vi "Process.vi"(8 "error in (no error)":errorcluster, 10 "Pound in":refnum<class "Pound.lvclass">, 11 "Qbus in":refnum<class "Qbus.lvclass">) -> (0 "error out":errorcluster)   [LabVIEW 2017, in "IrManageCameras.lvlib"]
uses:
  <vilib>/addons/InsightCM/Devices/Shared/Ir/IrManageCameras/IrManageCameras.lvlib
  <vilib>/addons/Qbus/Qbus.lvclass
  <vilib>/NI/Software Watchdog/Pound/Pound.lvclass
  <vilib>/addons/InsightCM/Devices/Shared/Ir/IrManageCameras/controls/config.ctl
  <vilib>/addons/InsightCM/Devices/Shared/Ir/IrManageCameras/controls/camera.ctl
  <vilib>/addons/TimerProcess/controls/taskType.ctl
  <vilib>/addons/TraceLogger/TraceLogger.lvlib
  <vilib>/NI/Software Watchdog/Watchdog/Watchdog.lvclass
  <vilib>/addons/SystemInfoProcess/SystemInfoProcess.lvlib
  <vilib>/addons/TimerProcess/TimerProcess.lvlib
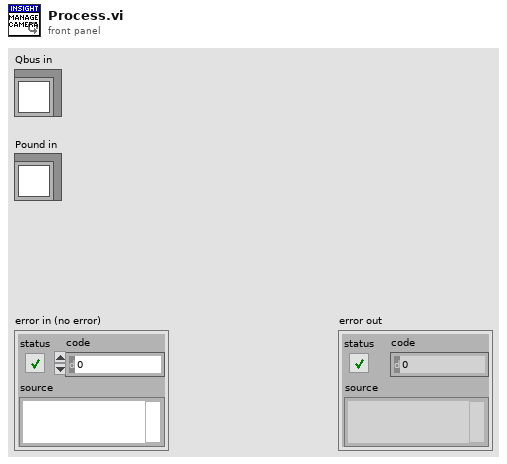
[diagram p1: front panel]
types:
  T1 = typedef "IrManageCameras.lvlib/config.ctl" = cluster{"discovered cameras":T2[]}
  T2 = typedef "IrManageCameras.lvlib/camera.ctl" = cluster{"InterfaceName":string, "VendorName":string, "ModelName":string, "CameraFileName":string, "SerialNumber":string, "IP Address":string, "PhysicalPort":string, "CameraName":string, "ChannelId":string, "CameraId":string, "InDeviceModel":bool}
  T3 = typedef "TimerProcess.lvlib/taskType.ctl" = enum16{"single", "repeat"}
  T4 = typedef "SystemInfoProcess.lvlib/NetworkAdapterSettings.ctl" = cluster{"Adapter Mode":u32, "IsPrimary":bool, "MACAddr":string, "IP Address Request Mode":u32, "IPAddr":string, "SubnetMask":string, "Gateway":string, "DNSServer":string, "Alias":string}
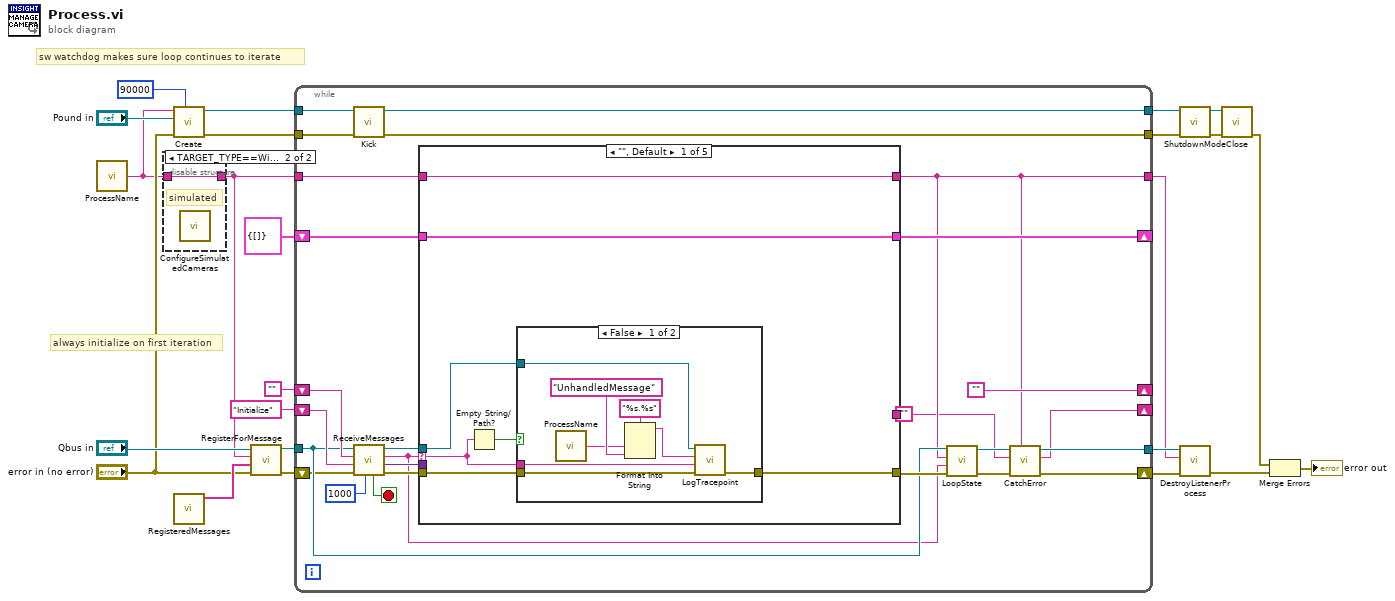
[diagram p0: block diagram]
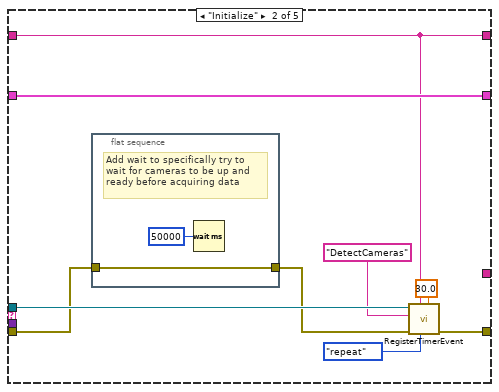
[diagram p4: hidden frame]
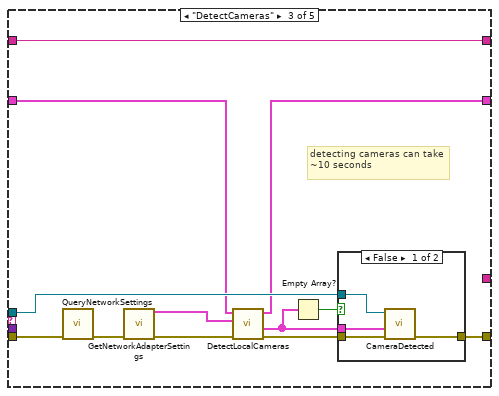
[diagram p5: hidden frame]
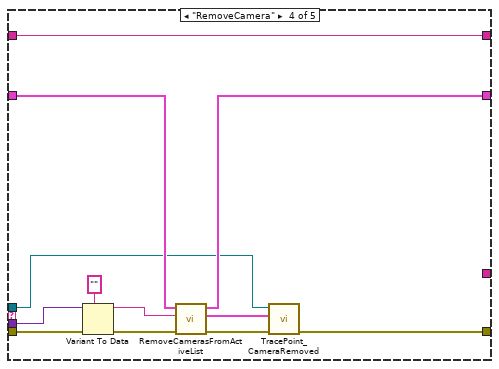
[diagram p7: hidden frame]
diagram:
  # "always initialize on first iteration"
  # "sw watchdog makes sure loop continues to iterate"
  n1 = call <vilib>:"ProcessName.vi"() -> ("process name"=w1:string)  [unwired: 5 in]
  n2 = disable-structure shown="TARGET_TYPE==Windows" {
    disable-tunnel: [w25 w26] -> w2
    disable-tunnel: w1 -> [w25 w26]
    frame condition #0 {
    }
    frame condition #1 (active) {
      # "simulated"
      n3 = call <vilib>:"ConfigureSimulatedCameras.vi"() -> ()  [unwired: 11 in, 1 out]
    }
  }
  n4 = call <vilib>:"Create.vi"("Execution Timeout (ms)"=u32 90000, "error in (no error)"="error in (no error)", "Pound"="Pound in", "Name"=w1) -> ("error out"=w8:errorcluster, "Watchdog"=w14:refnum<data-value>)  [unwired: 6 in]
  n5 = call <vilib>:"RegisteredMessages.vi"() -> ("registered messages"=w15:string[])  [unwired: 11 in]
  n6 = call <vilib>:"RegisterForMessage.vi"("error in (no error)"="error in (no error)", "message names"=w15, "process name"=w2, "Qbus in"="Qbus in") -> ("error in (no error)"=w23:errorcluster, "Qbus out"=w22:refnum<class "Qbus.lvclass">)  [unwired: 6 in]
  n7 = while {
    shift-right: [""] -> _
    shift-left: "" -> [w51]
    tunnel: w22 -> [w39]
    tunnel: w2 -> [w29]
    tunnel: [w42] -> w20
    tunnel: [w28] -> w19
    shift-right: [w41] -> _
    shift-left: "Initialize" -> [w46]
    shift-right: [w44] -> _
    shift-left: T1 {"discovered cameras"=[]} ("config") -> [w45]
    tunnel: w14 -> [w38]
    tunnel: [w37] -> w10
    tunnel: w8 -> [w36]
    tunnel: [w34] -> w7
    shift-right: [w43] -> w21
    shift-left: w23 -> [w35]
    stop <- w52 stop-if-true
    n8 = call <vilib>:"Kick.vi"("error in (no error)"=w36, "Watchdog"=w38) -> ("error out"=w34:errorcluster, "Watchdog"=w37:refnum<data-value>)  [unwired: 8 in]
    n9 = call <vilib>:"ReceiveMessages.vi"("Timeout(1000)"=1000 ("milliseconds to wait"), "error in (no error)"=w35, "priority action"=w46, "default action"=w51, "Qbus in"=w39) -> ("error out"=w50:errorcluster, "message value"=w47:variant, "action"=w33:string, "Qbus out"=w48:refnum<class "Qbus.lvclass">, "exit"=w52:bool)  [unwired: 2 in]
    n10 = case shown="\"\", Default" w33 {
      selector: w33 -> [w56 _ _ _ _]
      tunnel: w50 -> [w58 w71 w86 w108 w112]
      tunnel: w48 -> [w54 w77 w87 w104 _]
      tunnel: [w57 w73 w88 w103 w112] -> w40
      tunnel: w47 -> [_ _ _ w107 _]
      tunnel: w45 -> [w60 w78 w85 w106 w111]
      tunnel: [w60 w78 w84 w105 w111] -> w44
      tunnel: [w59 w76 w92 w109 w110] -> w28
      tunnel: w29 -> [w59 w76 w92 w109 w110]
      tunnel: ["" _ _ _ _] -> w27
      frame "", Default {
        n11 = Empty String/Path?(string/path=w56) -> (empty?=w55:bool)
        n12 = case shown="False" w55 {
          tunnel: [w64 w69] -> w57
          tunnel: w58 -> [w65 w69]
          tunnel: w56 -> [w62 _]
          tunnel: w54 -> [w63 _]
          frame False {
            n13 = call <vilib>:"ProcessName.vi"() -> ("process name"=w66:string)  [unwired: 5 in]
            n14 = Format Into String(format string="%s.%s", w66, "UnhandledMessage" ("ProcessName")) -> (resulting string=w61:string)  [unwired: 2 in, 1 out]
            n15 = call <vilib>:"LogTracepoint.vi"("error in (no error)"=w65, "log string"=w62, "tracepoint"=w61, "qbus in"=w63) -> ("error out"=w64:errorcluster)  [unwired: 6 in, 1 out]
          }
          frame True {
          }
        }
      }
      frame "Initialize" {
        n16 = flat-sequence {
          tunnel: w71 -> [w80]
          tunnel: [w80] -> w70
          frame #0 {
            # "Add wait to specifically try to\nwait for cameras to be up and \nready before acquiring data"
            n17 = Wait (ms)(milliseconds to wait=u32 50000) -> ()  [unwired: 1 out]
          }
        }
        n18 = call <vilib>:"RegisterTimerEvent.vi"("interval (sec)"=30.0, "type"=taskType."repeat", "process name"=w76, "error in (no error)"=w70, "callback action"="DetectCameras", "qbus in"=w77) -> ("error out"=w73:errorcluster)  [unwired: 4 in, 1 out]
      }
      frame "DetectCameras" {
        # "detecting cameras can take ~10 seconds"
        n19 = call <vilib>:"QueryNetworkSettings.vi"("error in (no error)"=w86) -> ("error out"=w91:errorcluster)  [unwired: 10 in]
        n20 = call <vilib>:"GetNetworkAdapterSettings.vi"("error in (no error)"=w91) -> ("error out"=w89:errorcluster, "Network Adapter Settings"=w90:T4[])  [unwired: 8 in, 1 out]
        n21 = call <vilib>:"DetectLocalCameras.vi"("error in (no error)"=w89, "network configuration"=w90, "config"=w85) -> ("error out"=w82:errorcluster, "new cameras"=w81:T2[], "config out"=w84:T1)  [unwired: 6 in]
        n22 = Empty Array?(array=w81) -> (empty?=w83:bool)
        n23 = case shown="False" w83 {
          tunnel: w82 -> [w96 w97]
          tunnel: [w94 w97] -> w88
          tunnel: w87 -> [w95 _]
          tunnel: w81 -> [w93 _]
          frame False {
            n24 = call <vilib>:"CameraDetected.vi"("error in (no error)"=w96, "new cameras"=w93, "Qbus in"=w95) -> ("error out"=w94:errorcluster)  [unwired: 8 in]
          }
          frame True {
            # "no new cameras"
          }
        }
      }
      frame "RemoveCamera" {
        n25 = Variant To Data(error in=w108, type="", Variant=w107) -> (data=w98:string, error out=w102:errorcluster)
        n26 = call <vilib>:"RemoveCamerasFromActiveList.vi"("error in (no error)"=w102, "camera to remove"=w98, "config"=w106) -> ("error out"=w100:errorcluster, "cameras removed"=w101:T2[], "config out"=w105:T1)  [unwired: 6 in]
        n27 = call <vilib>:"TracePoint_CameraRemoved.vi"("error in (no error)"=w100, "cameras removed"=w101, "Qbus"=w104) -> ("error out"=w103:errorcluster)  [unwired: 8 in]
      }
      frame "Exit" {
      }
    }
    n28 = call <vilib>:"LoopState.vi"("error in (no error)"=w40, "loop action"=w33, "process name"=w28, "Qbus in"=w39) -> ("error out"=w31:errorcluster, "Qbus out"=w30:refnum<class "Qbus.lvclass">)  [unwired: 6 in]
    n29 = call <vilib>:"CatchError.vi"("source"=w28, "error in (no error)"=w31, "next action in"=w27, "Qbus in"=w30) -> ("error out"=w43:errorcluster, "next action out"=w41:string, "Qbus out"=w42:refnum<class "Qbus.lvclass">)  [unwired: 5 in]
  }
  n30 = call <vilib>:"ShutdownMode.vi"("error in (no error)"=w7, "Watchdog"=w10) -> ("error out"=w9:errorcluster, "Watchdog"=w11:refnum<data-value>)  [unwired: 8 in]
  n31 = call <vilib>:"DestroyListenerProcess.vi"("error in (no error)"=w21, "process name"=w19, "Qbus in"=w20) -> ("error in (no error)"=w6:errorcluster)  [unwired: 7 in, 1 out]
  n32 = call <vilib>:"Close.vi"("error in (no error)"=w9, "Watchdog"=w11) -> ("error out"=w5:errorcluster)  [unwired: 9 in]
  n33 = Merge Errors(w5, w6) -> (→"error out":errorcluster)
